vi "Write TestLimitPath.vi"(8 "error in (no error)":errorcluster, 10 "TestLimitPath":path, 11 "TestSetup in":refnum<class "TestSetup.lvclass">) -> (0 "error out":errorcluster, 3 "TestSetup out":refnum<class "TestSetup.lvclass">)   [LabVIEW 2019, in "TestSetup.lvlib" / "TestSetup.lvclass"]
uses:
  TestSetup.lvclass
  TestSetup.lvclass/TestSetup.ctl
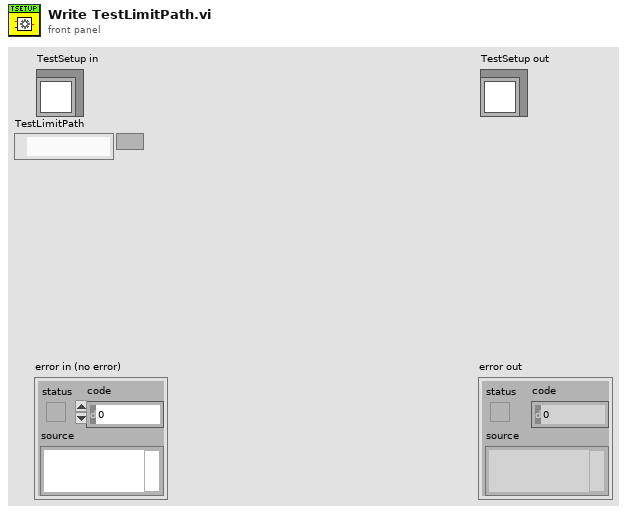
[diagram p1: front panel]
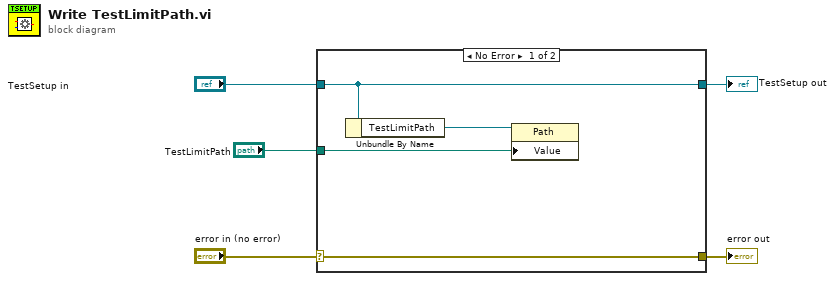
[diagram p0: block diagram]
diagram:
  n1 = case shown="No Error" "error in (no error)" {
    selector: "error in (no error)" -> [w9 w10]
    tunnel: [w9 w10] -> w4
    tunnel: [w8 w11] -> w2
    tunnel: "TestSetup in" -> [w8 w11]
    tunnel: "TestLimitPath" -> [w6 _]
    frame No Error {
      n2 = Unbundle By Name(w8) -> ("TestLimitPath"=w7:refnum<vi>)
      n3 = property class="Path"(reference=w7, "Value"=w6) -> ()  [unwired: 1 in, 2 out]
    }
    frame Error {
    }
  }
  "error out" <- w4
  "TestSetup out" <- w2
